vi "Solve1.vi"(8 "Error In":errorcluster, 11 "object in":refnum<class "2021_13.lvclass">) -> (0 "Error Out":errorcluster, 2 "Result":u64, 3 "object out":refnum<class "2021_13.lvclass">)   [LabVIEW 2020, in "2021_13.lvclass"]
uses:
  2021_13.lvclass
  2021_13.lvclass/2021_13.ctl
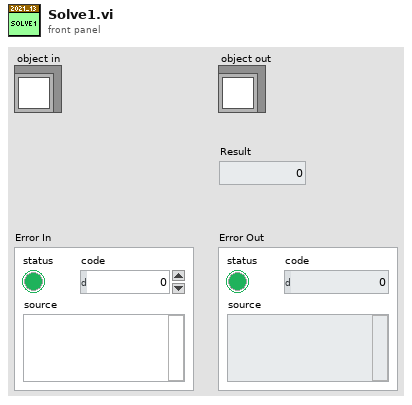
[diagram p1: front panel]
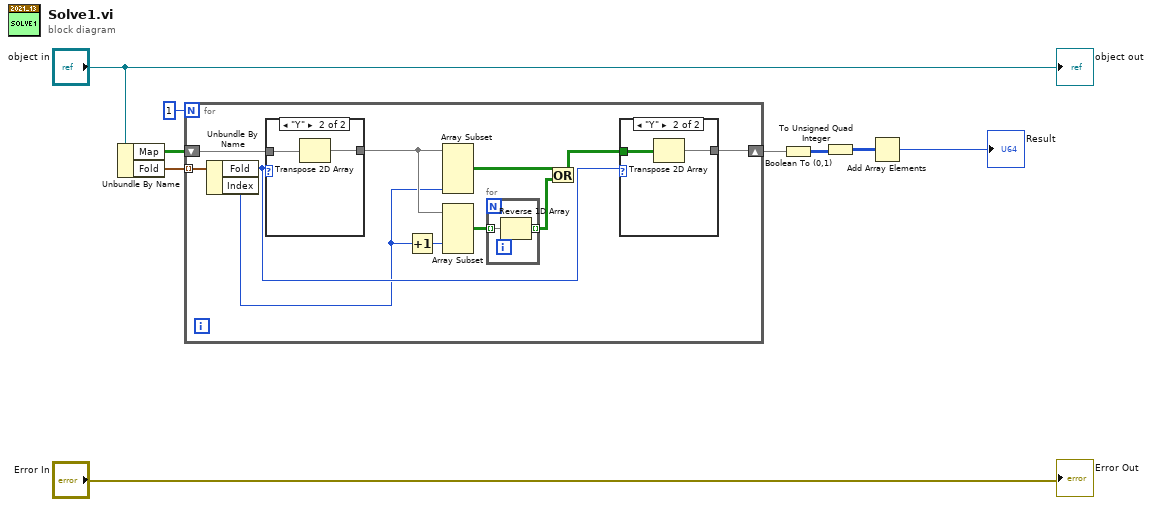
[diagram p0: block diagram]
diagram:
  n1 = Unbundle By Name("object in") -> ("Map"=w6:bool[][], "Fold"=w7:cluster{"Fold":enum16{"X", "Y"}, "Index":i32}[])
  n2 = for {
    N: 1 -> [_]
    tunnel: w7 -> [w20] mode=indexing
    shift-right: [w10] -> w5
    shift-left: w6 -> [w19]
    n3 = Unbundle By Name(w20) -> ("Fold"=w18:enum16{"X", "Y"}, "Index"=w16:i32)
    n4 = case shown="\"Y\"" w18 {
      tunnel: w19 -> [w26 w28]
      tunnel: [w26 w27] -> w17
      frame "X", Default {
      }
      frame "Y" {
        n5 = Transpose 2D Array(2D array=w28) -> (transposed array=w27:bool[][])
      }
    }
    n6 = Increment(x=w16) -> (x+1=w15:i32)
    n7 = Array Subset(array=w17, length (col)=w16) -> (w13:bool[][])  [unwired: 3 in]
    n8 = Array Subset(array=w17, index (col)=w15) -> (w14:bool[][])  [unwired: 3 in]
    n9 = for {
      tunnel: w14 -> [w22] mode=indexing
      tunnel: [w21] -> w12 mode=indexing
      n10 = Reverse 1D Array(array=w22) -> (reversed array=w21:bool[])
    }
    n11 = Or(x=w13, y=w12) -> (x .or. y?=w11:bool[][])
    n12 = case shown="\"Y\"" w18 {
      tunnel: w11 -> [w23 w25]
      tunnel: [w23 w24] -> w10
      frame "X", Default {
      }
      frame "Y" {
        n13 = Transpose 2D Array(2D array=w25) -> (transposed array=w24:bool[][])
      }
    }
  }
  n14 = Boolean To (0,1)(Boolean=w5) -> (0, 1=w4:i16[][])
  n15 = To Unsigned Quad Integer(1:w4) -> (0:w3:u64[][])
  n16 = Add Array Elements(numeric array=w3) -> (sum=→"Result":u64)
  "Error Out" <- "Error In"
  "object out" <- "object in"
